vi "PROXY_read_config_files_to_fgv.vi"(6 "number_of_stations":i32, 8 "error_in":errorcluster, 11 "all_config_info_in":T1) -> (0 "error_out":errorcluster, 3 "all_config_info_out":T1)   [LabVIEW 2020]
uses:
  typedef/PROXY_all_config_info.ctl
  typedef/PROXY_main_ini_file.ctl
  queues/typedef/PROXY_queue_refnums.ctl
  queues/typedef/STATION_queue_element.ctl
  STATION/ST_SQL_sequence_state.ctl
  FGV/main_ini/FGV_PROXY_config_info.ctl
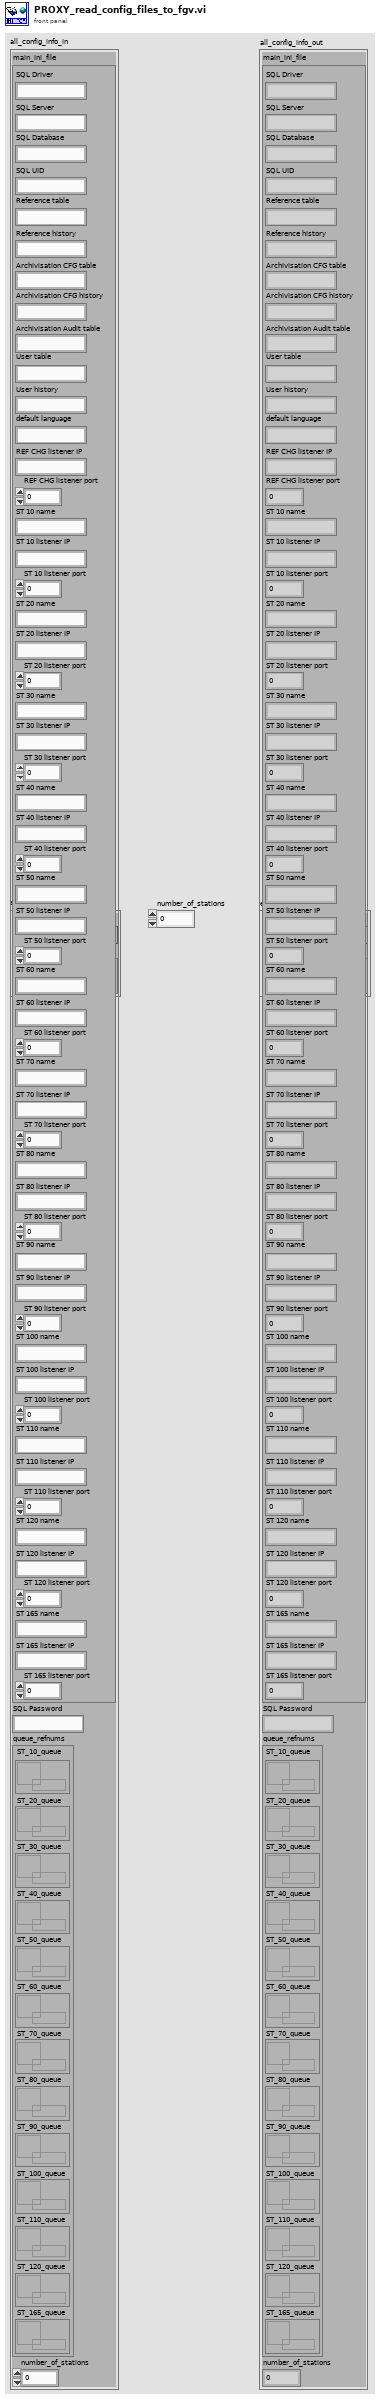
[diagram p1: front panel]
types:
  T1 = typedef "PROXY_all_config_info.ctl" = cluster{"main_ini_file":T2, "SQL Password":string, "queue_refnums":T3, "number_of_stations":i32}
  T2 = typedef "PROXY_main_ini_file.ctl" = cluster{"SQL Driver":string, "SQL Server":string, "SQL Database":string, "SQL UID":string, "Reference table":string, "Reference history":string, "Archivisation CFG table":string, "Archivisation CFG history":string, "Archivisation Audit table":string, "User table":string, "User history":string, "default language":string, "REF CHG listener IP":string, "REF CHG listener port":u16, "ST 10 name":string, "ST 10 listener IP":string, "ST 10 listener port":u16, "ST 20 name":string, "ST 20 listener IP":string, "ST 20 listener port":u16, "ST 30 name":string, "ST 30 listener IP":string, "ST 30 listener port":u16, "ST 40 name":string, "ST 40 listener IP":string, "ST 40 listener port":u16, "ST 50 name":string, "ST 50 listener IP":string, "ST 50 listener port":u16, "ST 60 name":string, "ST 60 listener IP":string, "ST 60 listener port":u16, "ST 70 name":string, "ST 70 listener IP":string, "ST 70 listener port":u16, "ST 80 name":string, "ST 80 listener IP":string, "ST 80 listener port":u16, "ST 90 name":string, "ST 90 listener IP":string, "ST 90 listener port":u16, "ST 100 name":string, "ST 100 listener IP":string, "ST 100 listener port":u16, "ST 110 name":string, "ST 110 listener IP":string, "ST 110 listener port":u16, "ST 120 name":string, "ST 120 listener IP":string, "ST 120 listener port":u16, "ST 165 name":string, "ST 165 listener IP":string, "ST 165 listener port":u16}
  T3 = typedef "PROXY_queue_refnums.ctl" = cluster{"ST_10_queue":refnum<queue>, "ST_20_queue":refnum<queue>, "ST_30_queue":refnum<queue>, "ST_40_queue":refnum<queue>, "ST_50_queue":refnum<queue>, "ST_60_queue":refnum<queue>, "ST_70_queue":refnum<queue>, "ST_80_queue":refnum<queue>, "ST_90_queue":refnum<queue>, "ST_100_queue":refnum<queue>, "ST_110_queue":refnum<queue>, "ST_120_queue":refnum<queue>, "ST_165_queue":refnum<queue>}
  T4 = typedef "FGV_PROXY_config_info.ctl" = enum16{"initialize", "set", "get"}
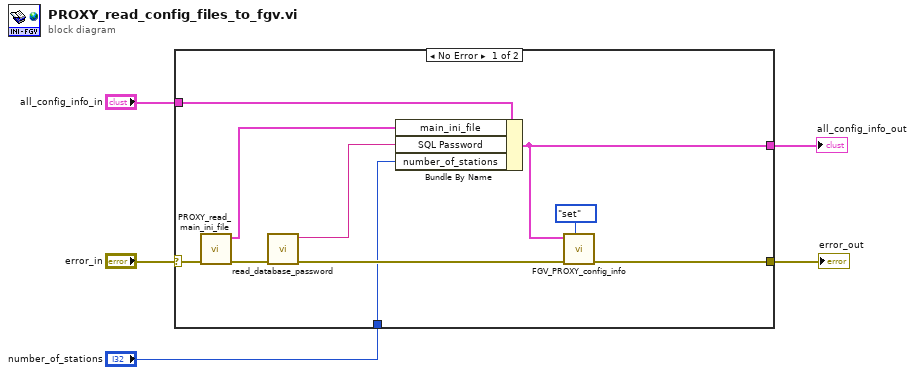
[diagram p0: block diagram]
diagram:
  n1 = case shown="No Error" "error_in" {
    selector: "error_in" -> [w15 w17]
    tunnel: [w7 w17] -> w5
    tunnel: [w6 w16] -> w1
    tunnel: "all_config_info_in" -> [w13 w16]
    tunnel: "number_of_stations" -> [w9 _]
    frame No Error {
      n2 = call "PROXY_read_main_ini_file.vi"("error_in"=w15) -> ("error_out"=w12:errorcluster, "main_ini_file_out"=w10:T2)  [unwired: 7 in, 2 out]
      n3 = call "read_database_password.vi"("error_in"=w12) -> ("error_out"=w11:errorcluster, "database_password"=w8:string)  [unwired: 8 in]
      n4 = Bundle By Name(cluster=w13, "main_ini_file"=w10, "SQL Password"=w8, "number_of_stations"=w9) -> (w6:T1)
      n5 = call "FGV_PROXY_config_info.vi"("options"=FGV_PROXY_config_info."set", "error_in"=w11, "all_config_info_in"=w6) -> ("error_out"=w7:errorcluster)  [unwired: 7 in, 1 out]
    }
    frame Error {
    }
  }
  "error_out" <- w5
  "all_config_info_out" <- w1
